vi "Fluke 28x Series Frequency Sweep.vi"() -> ()   [LabVIEW 2015]
doc: "This example shows how to configure and enable a frequency sweep."
uses:
  <instrlib>/Fluke 28x Series/Fluke 28x Series.lvlib
panel:
  in  "Sweep Marker (100 Hz)":dbl=100.0
  in  "Sweep Type (0: Continuous)":u16(ring) items=["Continuous", "Triggered", "Triggered, Hold/Reset"]
  in  "Sweep Spacing (0: Linear)":u16(ring) items=["Linear", "Log"]
  in  "Sweep Time (1.00 s)":dbl=1.0 format="%#.6g"
  in  "Start Frequency (100.0 Hz)":dbl=100.0 format="%#.6g"
  in  "Stop  Frequency  (1000.0 Hz)":dbl=1000.0 format="%#.6f"
  in  "Frequency (1000 Hz)":dbl=1000.0
  in  "Waveform Function (0: Sine)":u16(ring) items=["Sine", "Square", "Triangle", "Cosine", "DC", "Positive Ramp", "Negative Ramp", "Haversine", "Havercosine", "Sine (x)/x"]
  in  "Amplitude (1.0 Vpp)":dbl=1.0
  in  "DC Offset (0.00 V)":dbl
  in  "VISA resource name":refnum<visa-resource-name>
  # "(c) 2009-2014 National Instruments.  ALL RIGHTS RESERVED."
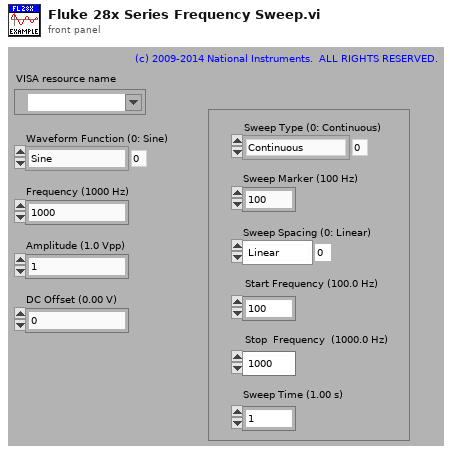
[diagram p1: front panel]
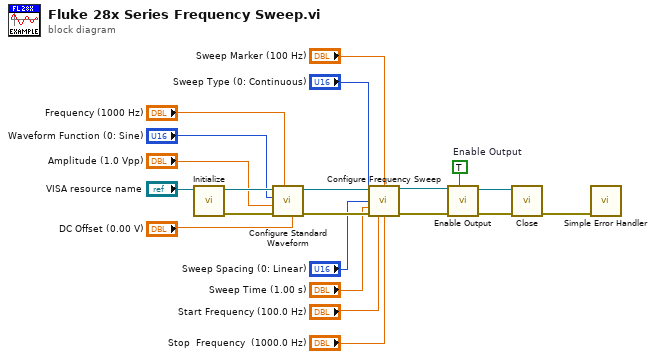
[diagram p0: block diagram]
diagram:
  w11 = TRUE  # Enable Output
  n1 = call <instrlib>:"Initialize.vi"("VISA resource name"="VISA resource name") -> ("error out"=w16:errorcluster, "VISA resource name out"=w21:refnum<visa-resource-name>)  [unwired: 9 in]
  n2 = call <instrlib>:"Configure Standard Waveform.vi"("DC Offset (0.00 V)"="DC Offset (0.00 V)", "Frequency (1000 Hz)"="Frequency (1000 Hz)", "error in (no error)"=w16, "Amplitude (1.0 Vpp)"="Amplitude (1.0 Vpp)", "Waveform Function (0: Sine)"="Waveform Function (0: Sine)", "VISA resource name"=w21) -> ("error out"=w19:errorcluster, "VISA resource name out"=w18:refnum<visa-resource-name>)  [unwired: 4 in]
  n3 = call <instrlib>:"Configure Frequency Sweep.vi"("VISA resource name"=w18, "Sweep Marker (100 Hz)"="Sweep Marker (100 Hz)", "Sweep Type (0: Continuous)"="Sweep Type (0: Continuous)", "Sweep Spacing (0: Linear)"="Sweep Spacing (0: Linear)", "Sweep Time (1.00 s)"="Sweep Time (1.00 s)", "error in (no error)"=w19, "Start Frequency (100.0 Hz)"="Start Frequency (100.0 Hz)", "Stop  Frequency  (1000.0 Hz)"="Stop  Frequency  (1000.0 Hz)") -> ("VISA resource name out"=w13:refnum<visa-resource-name>, "error out"=w12:errorcluster)  [unwired: 6 in]
  n4 = call <instrlib>:"Enable Output.vi"("Enable Output (T: Enable)"=w11, "error in (no error)"=w12, "VISA resource name"=w13) -> ("error out"=w15:errorcluster, "VISA resource name out"=w14:refnum<visa-resource-name>)  [unwired: 7 in]
  n5 = call <instrlib>:"Close.vi"("error in (no error)"=w15, "VISA resource name"=w14) -> ("error out"=w20:errorcluster)  [unwired: 9 in]
  n6 = call <vilib>:"Simple Error Handler.vi"("error in (no error)"=w20) -> ()  [unwired: 4 in, 5 out]
